vi "send_internal_trigger.vi"(7 "ensure unique insertion?":bool, 8 "error in":errorcluster, 10 "trigger":T1, 11 "ScanModeDL091001Scaffold in":refnum<class "ImagingModeDL091001Scaffold.lvclass">) -> (0 "error out":errorcluster, 3 "ScanModeDL091001Scaffold out":refnum<class "ImagingModeDL091001Scaffold.lvclass">)   [LabVIEW 2010, in "ImagingModeDL091001Scaffold.lvclass"]
uses:
  ImagingModeDL091001Scaffold.lvclass
  internal_triggers_enum.ctl
  common/classes/GenericToplevelComponent/GenericToplevelComponent/trigger_type_enum.ctl
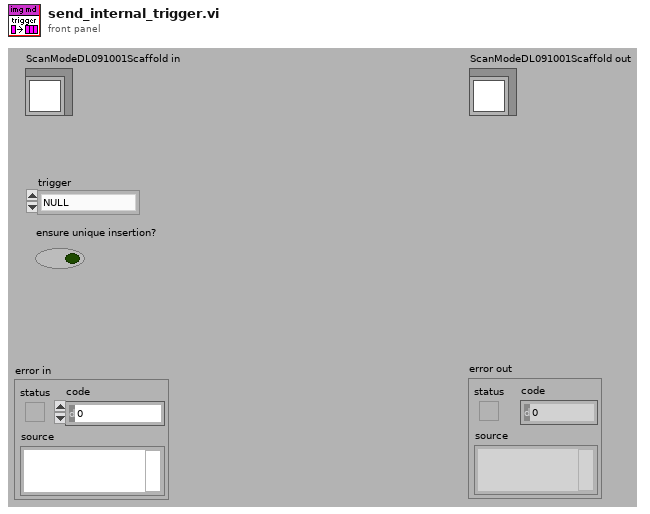
[diagram p1: front panel]
types:
  T1 = typedef "ImagingModeDL091001Scaffold.lvclass/internal_triggers_enum.ctl" = enum16{"NULL", "initialise", "terminate", "start sweep", "stop sweep", "update", "proceed", "draw overlay", "attach observer", "detach observer", "finish sweep"}
  T2 = typedef "trigger_type_enum.ctl" = enum8{"external", "internal", "common"}
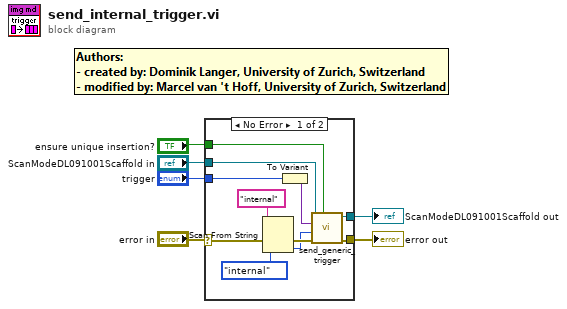
[diagram p0: block diagram]
diagram:
  n1 = case shown="No Error" "error in" {
    selector: "error in" -> [w11 w19]
    tunnel: [w13 w19] -> w2
    tunnel: [w14 w18] -> w3
    tunnel: "ScanModeDL091001Scaffold in" -> [w15 w18]
    tunnel: "ensure unique insertion?" -> [w16 _]
    tunnel: "trigger" -> [w17 _]
    frame No Error {
      n2 = Scan From String(input string="internal", error in=w11, default 1=trigger_type_enum."internal" ("trigger type")) -> (error out=w10:errorcluster, output 1=w8:T2)  [unwired: 2 in, 2 out]
      n3 = To Variant(anything=w17) -> (Variant=w12:variant)
      n4 = call-dynamic "send_generic_trigger.vi"("ensure unique insertion?"=w16, "error in (no error)"=w10, "trigger type"=w8, "trigger variant"=w12, "GenericToplevelComponent in"=w15) -> ("error out"=w13:errorcluster, "GenericToplevelComponent out"=w14:refnum<class "ImagingModeDL091001Scaffold.lvclass">)  [unwired: 3 in, 2 out]
    }
    frame Error {
    }
  }
  "error out" <- w2
  "ScanModeDL091001Scaffold out" <- w3
